vi "Get List of Map Providers.vi"(8 "Error In":errorcluster) -> (0 "error out":errorcluster, 2 "Array of Map Provider Refs":refnum<k24>[](array[refnum]), 3 "Array of Map Provider Names":string[](array[string]))   [LabVIEW 2014]
uses:
  C:/Robotic Systems/Products/AgFalcon/Software/Ground Station/Data/Mapping DLL/GMap.NET.Core.dll
  Data/Mapping DLL/GMap.NET.Core.dll
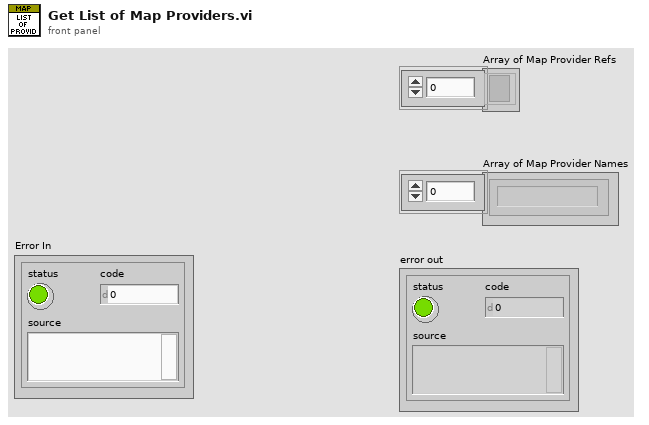
[diagram p1: front panel]
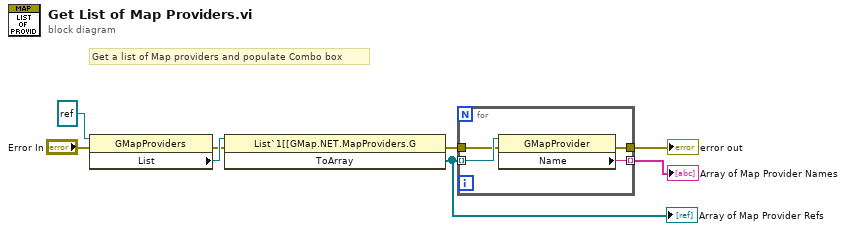
[diagram p0: block diagram]
diagram:
  # "Get a list of Map providers and populate Combo box"
  n1 = property class="GMapProviders"(reference=refnum<k24> refnum, error in="Error In") -> (error out=w4:errorcluster, "List"=w8:refnum<k24>)  [unwired: 1 out]
  n2 = invoke class="List`1[[GMap.NET.MapProviders.G" method="ToArray"(reference=w8, error in=w4) -> (error out=w7:errorcluster, "ToArray"=w3:refnum<k24>[])  [unwired: 1 in, 1 out]
  "Array of Map Provider Refs" <- w3
  n3 = for {
    tunnel: w3 -> [w12] mode=indexing
    tunnel: [w11] -> w1 mode=indexing
    tunnel: [w9] -> w2
    tunnel: w7 -> [w10]
    n4 = property class="GMapProvider"(reference=w12, error in=w10) -> (error out=w9:errorcluster, "Name"=w11:string)  [unwired: 1 out]
  }
  "error out" <- w2
  "Array of Map Provider Names" <- w1
